vi "countExistingGoals.vi"(8 "error in (no error)":errorcluster, 10 "WhichMonth.lvclass":refnum<class "WhichMonth.lvclass">, 11 "Account History in":refnum<class "Account History.lvclass">) -> (0 "error out":errorcluster, 2 "Goal  Count":i32, 3 "Account History out":refnum<class "Account History.lvclass">)   [LabVIEW 2018, in "Account History.lvclass"]
uses:
  Account History.lvclass
  WhichMonth/WhichMonth.lvclass
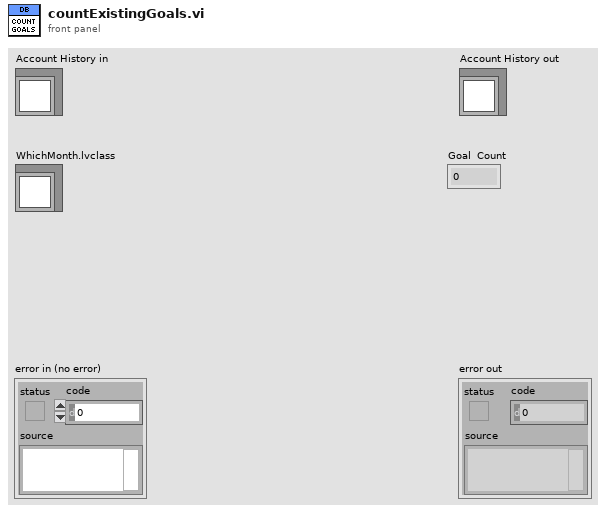
[diagram p1: front panel]
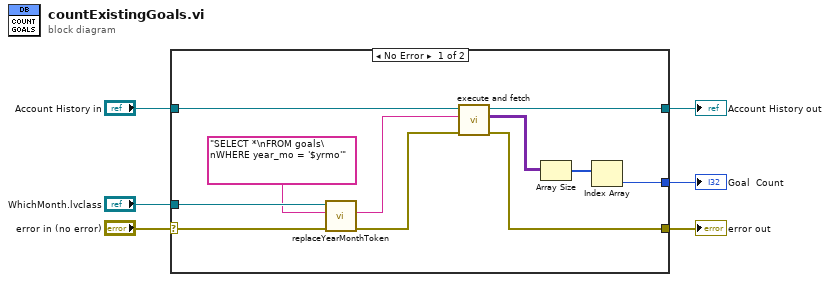
[diagram p0: block diagram]
diagram:
  n1 = case shown="No Error" "error in (no error)" {
    selector: "error in (no error)" -> [w15 w19]
    tunnel: [w8 w19] -> w5
    tunnel: [w11 w18] -> w3
    tunnel: "Account History in" -> [w14 w18]
    tunnel: "WhichMonth.lvclass" -> [w17 _]
    tunnel: [w7 _] -> w1
    frame No Error {
      n2 = call "replaceYearMonthToken.vi"("error in (no error)"=w15, "Query In"="SELECT *\nFROM goals\nWHERE year_mo = '$yrmo'", "WhichMonth in"=w17) -> ("error out"=w13:errorcluster, "Query Out"=w12:string)  [unwired: 6 in, 1 out]
      n3 = call "execute and fetch.vi"("error in (no error)"=w13, "SQL query"=w12, "Database in"=w14) -> ("error out"=w8:errorcluster, "recordset data"=w9:variant[][], "Database out"=w11:refnum<class "Account History.lvclass">)  [unwired: 5 in, 1 out]
      n4 = Array Size(array=w9) -> (size(s)=w10:i32[])
      n5 = Index Array(array=w10) -> (element=w7:i32)  [unwired: 1 in]
    }
    frame Error {
    }
  }
  "error out" <- w5
  "Account History out" <- w3
  "Goal  Count" <- w1
